vi "openQueue.vi"(8 "error in (no error)":errorcluster, 9 "Exclusive":bool=TRUE, 10 "Queue Name In":string, 11 "RabbitMQ Session In":T1) -> (0 "error out":errorcluster, 2 "Queue Name out":string, 3 "RabbitMQ Session Out":T1)   [LabVIEW 2019, in "rabbitmq.lvlib"]
uses:
  rabbitmq.lvlib
  session.ctl
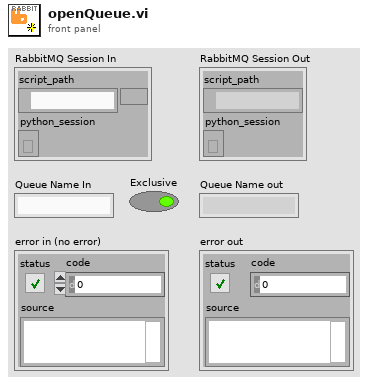
[diagram p1: front panel]
types:
  T1 = typedef "rabbitmq.lvlib/session.ctl" = cluster{"script_path":path, "python_session":refnum<k35>}
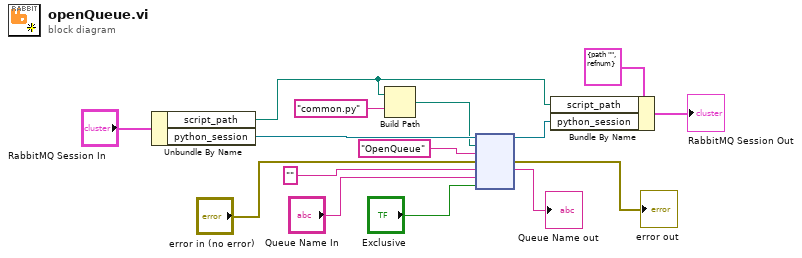
[diagram p0: block diagram]
diagram:
  n1 = Unbundle By Name("RabbitMQ Session In") -> ("script_path"=w5:path, "python_session"=w10:refnum<k35>)
  n2 = Build Path(base path=w5, name or relative path="common.py") -> (appended path=w4:path)
  n3 = node(w10, w4, "OpenQueue" ("function name"), "error in (no error)", "", "Queue Name In", "Exclusive") -> (w14:refnum<k35>, →"error out":errorcluster, →"Queue Name out":string)  [unwired: 2 in, 2 out]
  n4 = Bundle By Name(cluster=T1 {"script_path"=path "", "python_session"=refnum}, "script_path"=w5, "python_session"=w14) -> (→"RabbitMQ Session Out":T1)
